vi "Tree.vi"   [LabVIEW 2014]
uses:
  GLue.lvlib
panel:
  # "menu->View->VI Hierarchy \nto view the VI relationships"
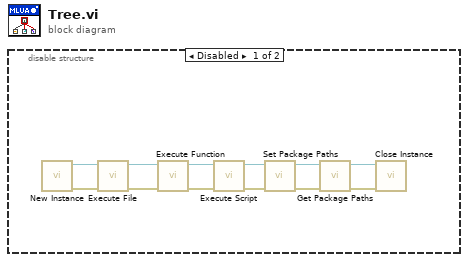
[diagram p0: block diagram]
diagram:
  n1 = disable-structure shown="Disabled" {
    frame Disabled {
      n2 = call "New Instance.vi"() -> ("error out"=w12:errorcluster, "GLue out"=w11:refnum<class "class.GLue.lvclass">)  [unwired: 10 in]
      n3 = call "Execute File.vi"("error in"=w12, "GLue in"=w11) -> ("error out"=w10:errorcluster, "GLue out"=w9:refnum<class "class.GLue.lvclass">)  [unwired: 7 in, 1 out]
      n4 = call "Execute Function.vi"("error in"=w10, "GLue in"=w9) -> ("error out"=w8:errorcluster, "GLue out"=w7:refnum<class "class.GLue.lvclass">)  [unwired: 7 in, 1 out]
      n5 = call "Execute Script.vi"("error in"=w8, "GLue in"=w7) -> ("error out"=w3:errorcluster, "GLue out"=w4:refnum<class "class.GLue.lvclass">)  [unwired: 7 in, 1 out]
      n6 = call "Set Package Paths.vi"("error in"=w3, "GLue in"=w4) -> ("error out"=w6:errorcluster, "GLue out"=w5:refnum<class "class.GLue.lvclass">)  [unwired: 8 in]
      n7 = call "Get Package Paths.vi"("GLue in"=w5, "error in"=w6) -> ("GLue out"=w2:refnum<class "class.GLue.lvclass">, "error out"=w1:errorcluster)  [unwired: 6 in, 2 out]
      n8 = call "Close Instance.vi"("error in"=w1, "GLue in"=w2) -> ()  [unwired: 9 in, 1 out]
    }
    frame Enabled {
    }
  }
